vi "Parsing_TheGoodOne.vi"(8 "Search_Params":string[](array[string])=["B", "X", "Y", "W1", "H1", "W2", "H2"], 9 "Input":string="B:2,X:197.00,Y:124.00,W1:9,H1:24,W2:9,H2:23") -> (2 "Corrected distance":dbl=59.99119999999999, 3 "Value-Reference":dbl=44.76553104454399)   [LabVIEW 2016]
panel:
  out "Positions 2":i32[](array[numeric])
  out "Distance":dbl=59.99119999999999
  out "Move left":bool
  out "Move right":bool
  out "Not target":bool=TRUE
  in  "Desired_Midpoint":i32=200
  in  "High_Band":i32=10
  in  "Low_Band":i32=10
  out "Error":i32
  in  "P-gain":dbl format="%#_13g"
  out "Effort_Error":dbl
  out "Good_Midp":bool
  out "X Value":i32=197
  out "Good Target 2":bool=TRUE
  out "Positions":i32[](array[numeric])
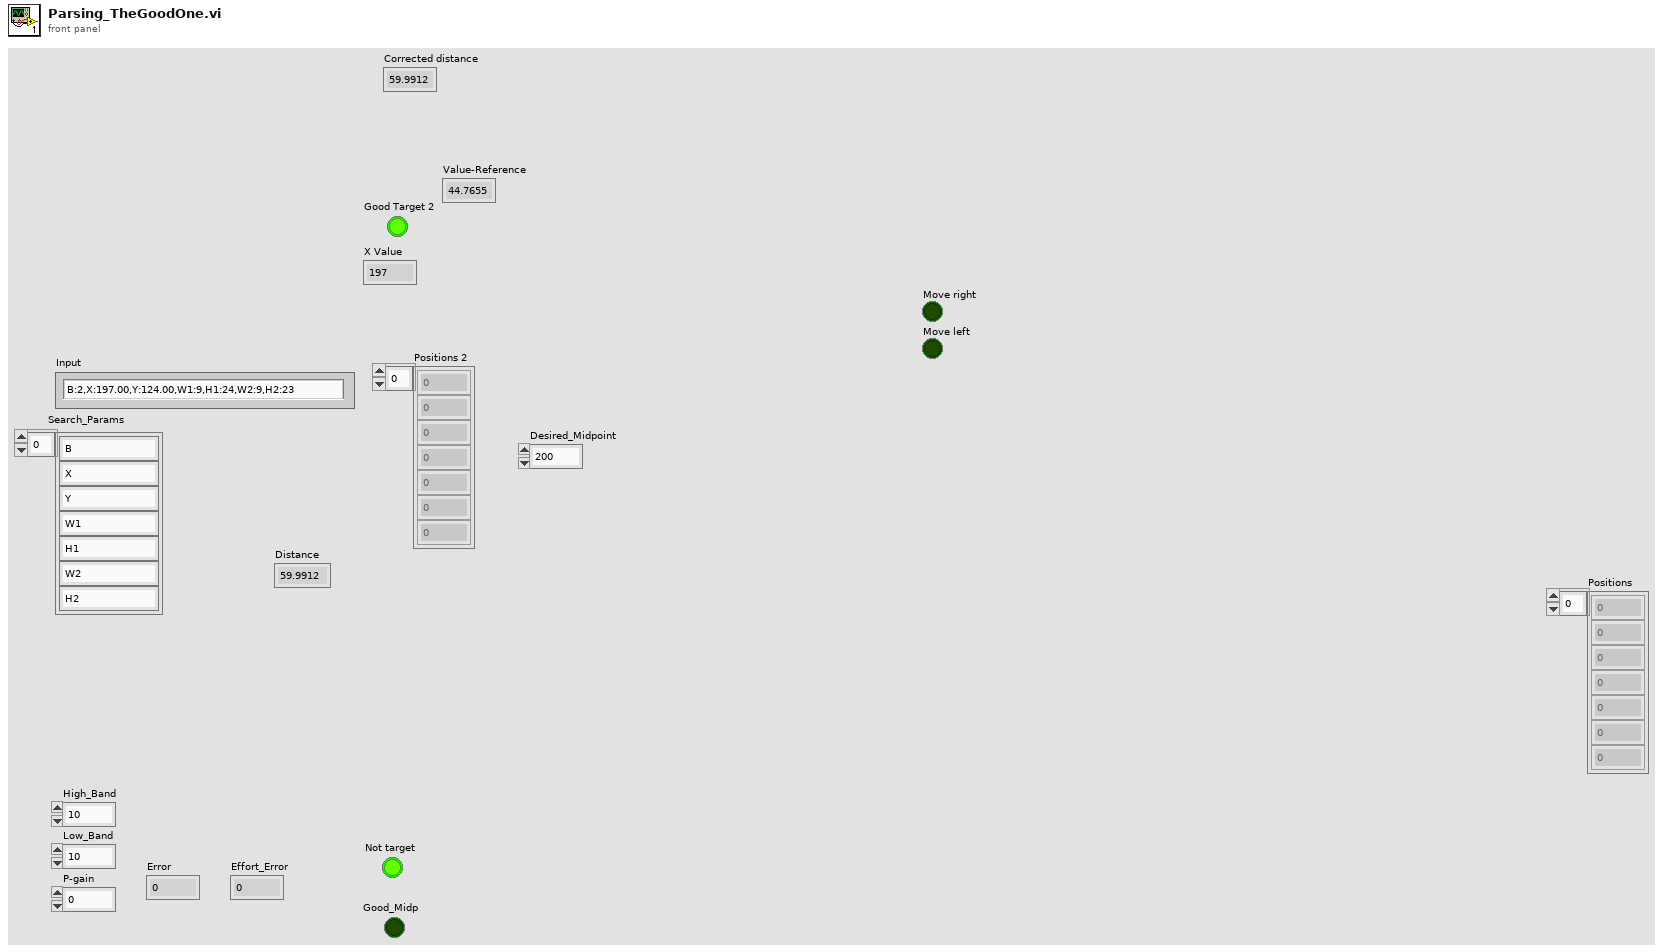
[diagram p1: front panel]
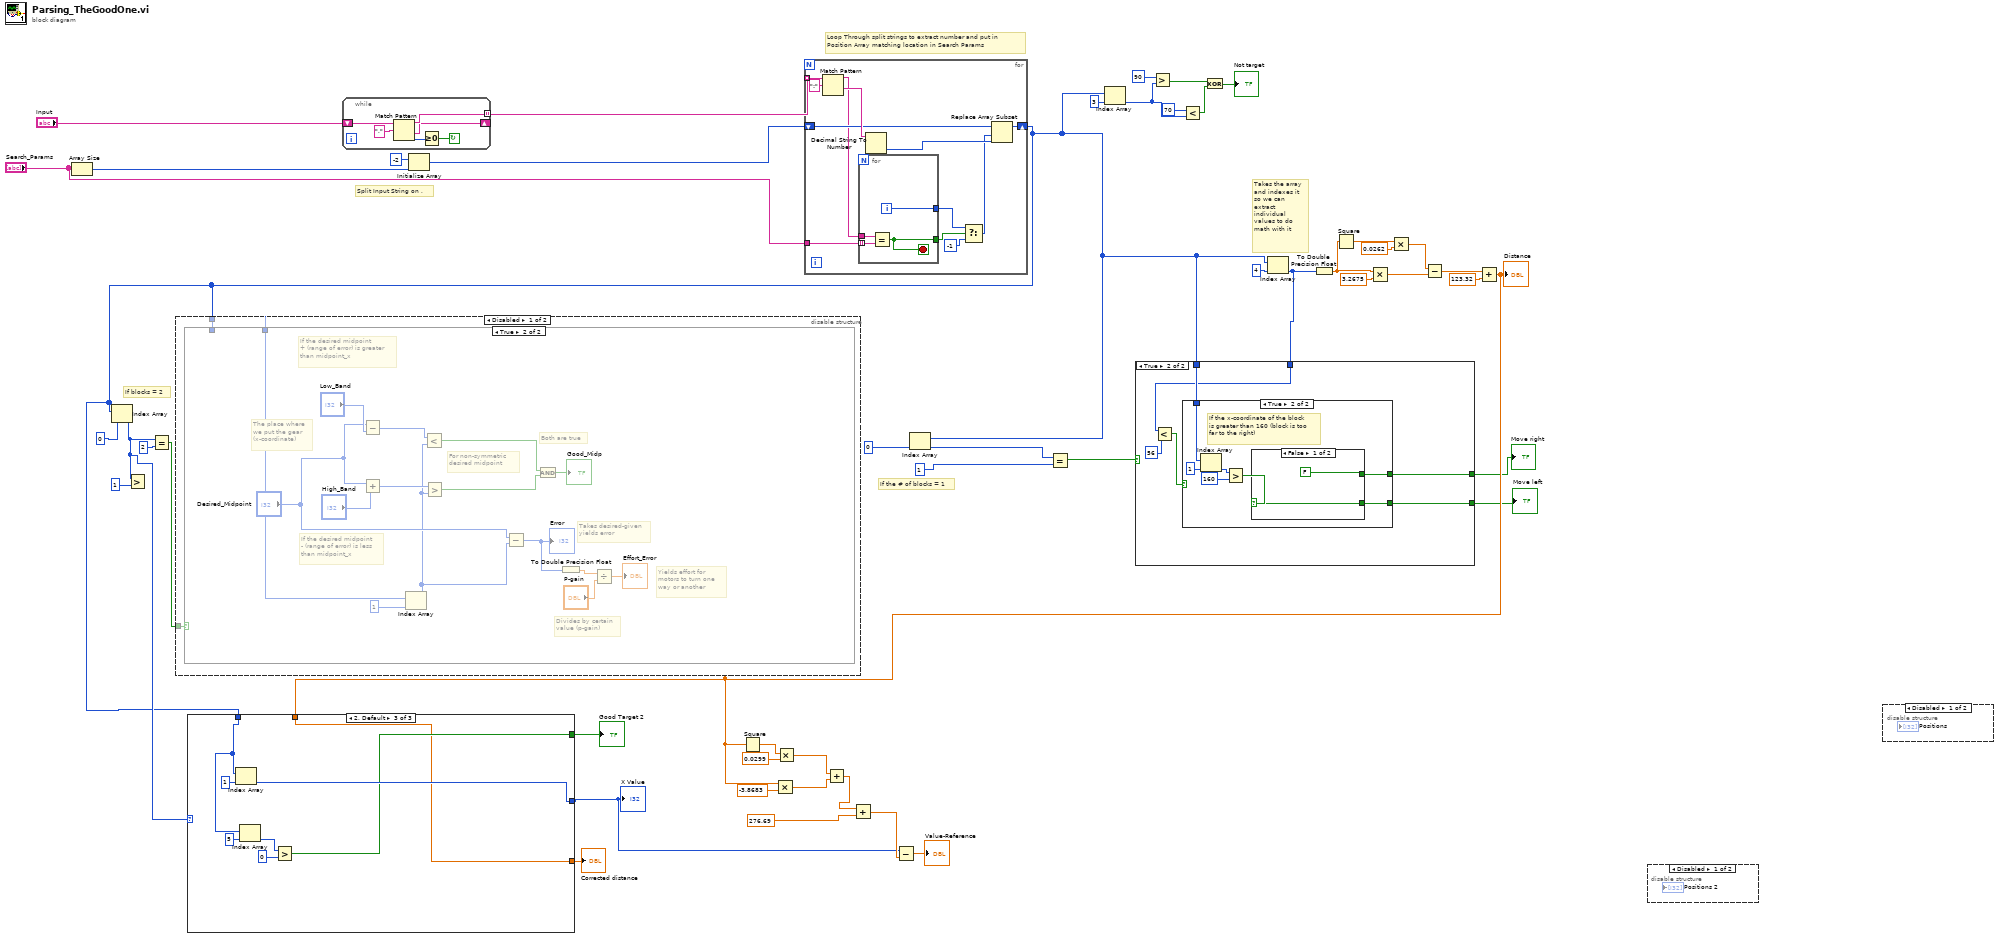
[diagram p0: block diagram]
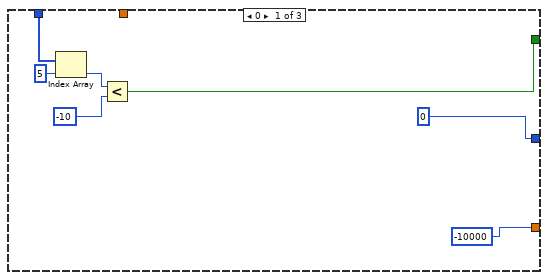
[diagram p2: hidden frame]
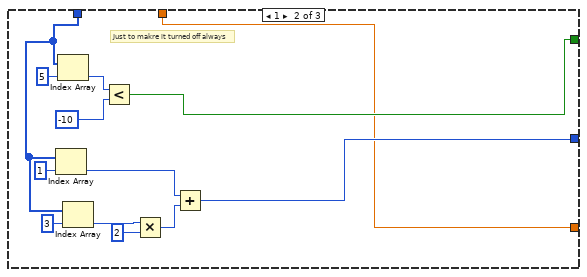
[diagram p3: hidden frame]
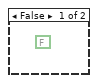
[diagram p4: hidden frame]
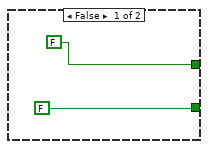
[diagram p6: hidden frame]
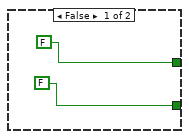
[diagram p7: hidden frame]
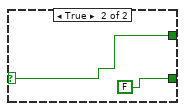
[diagram p8: hidden frame]
diagram:
  # "If blocks = 2"
  # "If the # of blocks = 1"
  # "Takes the array and indexes it so we can extract individual values to do math with it"
  # "Loop Through split strings to extract number and put in\nPosition Array matching location in Search Params"
  # "Split Input String on ,"
  n1 = Array Size(array="Search_Params") -> (size(s)=w7:i32)
  n2 = while {
    shift-right: [w51] -> _
    shift-left: "Input" -> [w54]
    tunnel: [w52] -> w3 mode=indexing
    stop <- w49 continue-if-true
    n3 = Match Pattern(string=w54, regular expression=",") -> (before substring=w52:string, after substring=w51:string, offset past match=w50:i32)  [unwired: 1 in, 1 out]
    n4 = Greater Or Equal To 0?(x=w50) -> (x >= 0?=w49:bool)
  }
  n5 = Initialize Array(-2 ("element"), w7) -> (w5:i32[])
  n6 = for {
    tunnel: w3 -> [w66] mode=indexing
    shift-right: [w62] -> w35
    shift-left: w5 -> [w63]
    tunnel: "Search_Params" -> [w59]
    n7 = Match Pattern(string=w66, regular expression=":") -> (before substring=w60:string, after substring=w64:string)  [unwired: 1 in, 2 out]
    n8 = for {
      tunnel: w60 -> [w70]
      tunnel: w59 -> [w69] mode=indexing
      tunnel: [w67] -> w58
      tunnel: [w68] -> w57
      i -> [w68]
      stop <- w67 stop-if-true
      n9 = Equal?(x=w70, y=w69) -> (x = y?=w67:bool)
    }
    n10 = Decimal String To Number(string=w64) -> (number=w61:i32)  [unwired: 2 in, 1 out]
    n11 = Select(t=w57, s=w58, f=-1) -> (s? t:f=w55:i32)
    n12 = Replace Array Subset(array=w63, new element=w61, index=w55) -> (w62:i32[])
  }
  n13 = Index Array(array=w35, index=0) -> (element=w36:i32)
  n14 = Greater?(x=w36, y=1) -> ()  [unwired: 1 out]
  n15 = Equal?(x=w36, y=2) -> (x = y?=w26:bool)
  n16 = disable-structure shown="Disabled" {
    disable-tunnel: w26 -> [w72 _]
    disable-tunnel: w35 -> [w71 _]
    frame Disabled {
      n17 = case shown="True" w72 {
        tunnel: w71 -> [_ _]
        tunnel: w71 -> [_ w73]
        frame False {
          (unwired) FALSE
        }
        frame True {
          # "Yields effort for\nmotors to turn one\nway or another"
          # "Divides by certain\nvalue (p-gain)"
          # "Takes desired-given\nyields error"
          # "The place where\nwe put the gear \n(x-coordinate)"
          # "Both are true"
          # "For non-symmetric\ndesired midpoint"
          # "If the desired midpoint\n- (range of error) is less\nthan midpoint_x"
          # "If the desired midpoint\n+ (range of error) is greater\nthan midpoint_x"
          n18 = Subtract(x="Desired_Midpoint", y="Low_Band") -> (x-y=w83:i32)
          n19 = Add(x="Desired_Midpoint", y="High_Band") -> (x+y=w84:i32)
          n20 = Index Array(array=w73, index=1) -> (element=w79:i32)
          n21 = Less?(x=w83, y=w79) -> (x < y?=w82:bool)
          n22 = Greater?(x=w84, y=w79) -> (0:w81:bool)
          n23 = Subtract(x="Desired_Midpoint", y=w79) -> (x-y=w78:i32)
          "Error" <- w78
          n24 = And(x=w82, y=w81) -> (x .and. y?=→"Good_Midp":bool)
          n25 = To Double Precision Float(number=w78) -> (double precision float=w77:dbl)
          n26 = Divide(x=w77, y="P-gain") -> (x/y=→"Effort_Error":dbl)
        }
      }
    }
    frame Enabled {
    }
  }
  n27 = Index Array(array=w35, index=0) -> (element=w18:i32)
  n28 = Equal?(x=w18, y=1) -> (x = y?=w20:bool)
  n29 = Index Array(array=w35, index=3) -> (element=w29:i32)
  n30 = Greater?(x=90, y=w29) -> (0:w31:bool)
  n31 = Less?(x=70, y=w29) -> (x < y?=w32:bool)
  n32 = Exclusive Or(1:w32, 2:w31) -> (0:→"Not target":bool)
  n33 = Index Array(array=w35, index=4) -> (element=w21:i32)
  n34 = case shown="True" w20 {
    tunnel: w35 -> [_ w95]
    tunnel: w21 -> [_ w93]
    tunnel: [FALSE w91] -> w22
    tunnel: [FALSE w90] -> w23
    frame False {
    }
    frame True {
      n35 = Less?(x=w93, y=56) -> (x < y?=w92:bool)
      n36 = case shown="True" w92 {
        tunnel: w95 -> [_ w104]
        tunnel: [FALSE w99] -> w91
        tunnel: [FALSE w98] -> w90
        frame False {
        }
        frame True {
          # "If the x-coordinate of the block\nis greater than 160 (block is too\nfar to the right)"
          n37 = Index Array(array=w104, index=1) -> (element=w102:i32)
          n38 = Greater?(x=w102, y=160) -> (0:w100:bool)
          n39 = case shown="False" w100 {
            selector: w100 -> [w106 w108]
            tunnel: [w106 FALSE] -> w99
            tunnel: [FALSE w108] -> w98
            frame False {
            }
            frame True {
            }
          }
        }
      }
    }
  }
  "Move left" <- w22
  "Move right" <- w23
  n40 = To Double Precision Float(number=w21) -> (double precision float=w11:dbl)
  n41 = Square(x=w11) -> (x^2=w9:dbl)
  n42 = Multiply(x=w11, y=3.2675) -> (x*y=w13:dbl)
  n43 = Multiply(x=w9, y=0.0262) -> (x*y=w10:dbl)
  n44 = Subtract(x=w10, y=w13) -> (x-y=w14:dbl)
  n45 = Add(x=w14, y=123.32) -> (x+y=w40:dbl)
  "Distance" <- w40
  n46 = case shown="2, Default" w36 {
    tunnel: w35 -> [w112 w124 w135]
    tunnel: w40 -> [_ w116 w129]
    tunnel: [0 w118 w131] -> w46
    tunnel: [w110 w117 w130] -> w37
    tunnel: [-10000 w116 w129] -> w1
    frame 0 {
      n47 = Index Array(array=w112, index=5) -> (element=w114:i32)
      n48 = Less?(x=w114, y=-10) -> (x < y?=w110:bool)
    }
    frame 1 {
      # "Just to makre it turned off always"
      n49 = Index Array(array=w124, index=1) -> (element=w119:i32)
      n50 = Index Array(array=w124, index=5) -> (element=w126:i32)
      n51 = Index Array(array=w124, index=3) -> (element=w122:i32)
      n52 = Less?(x=w126, y=-10) -> (x < y?=w117:bool)
      n53 = Multiply(x=w122, y=2) -> (x*y=w120:i32)
      n54 = Add(x=w119, y=w120) -> (x+y=w118:i32)
    }
    frame 2, Default {
      n55 = Index Array(array=w135, index=1) -> (element=w131:i32)
      n56 = Index Array(array=w135, index=5) -> (element=w133:i32)
      n57 = Greater?(x=w133, y=0) -> (0:w130:bool)
    }
  }
  "X Value" <- w46
  "Good Target 2" <- w37
  "Corrected distance" <- w1
  n58 = Square(x=w40) -> (x^2=w38:dbl)
  n59 = Multiply(x=w40, y=-3.8683) -> (x*y=w43:dbl)
  n60 = Multiply(x=w38, y=0.0299) -> (x*y=w42:dbl)
  n61 = Add(x=w42, y=w43) -> (x+y=w45:dbl)
  n62 = Add(x=w45, y=276.69) -> (x+y=w47:dbl)
  n63 = Subtract(x=w46, y=w47) -> (x-y=→"Value-Reference":dbl)
  n64 = disable-structure shown="Disabled" {
    frame Disabled {
    }
    frame Enabled {
    }
  }
  n65 = disable-structure shown="Disabled" {
    frame Disabled {
    }
    frame Enabled {
    }
  }
